vi "Read Session.vi"(8 "error in (no error)":errorcluster, 11 "Fgen PXI CFG in":refnum<class "Fgen PXI CFG.lvclass">) -> (0 "error out":errorcluster, 2 "Session":refnum<k15>, 3 "Fgen PXI CFG out":refnum<class "Fgen PXI CFG.lvclass">)   [LabVIEW 2023, in "Fgen PXI.lvlib" / "Fgen PXI CFG.lvclass"]
uses:
  Fgen PXI CFG.lvclass
  Fgen PXI CFG.lvclass/Fgen PXI CFG.ctl
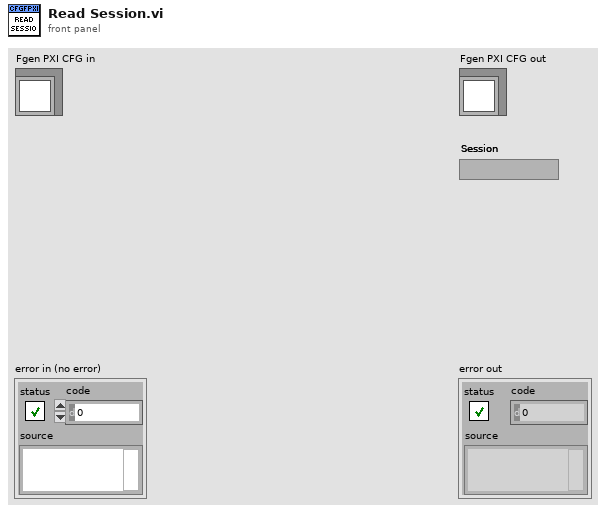
[diagram p1: front panel]
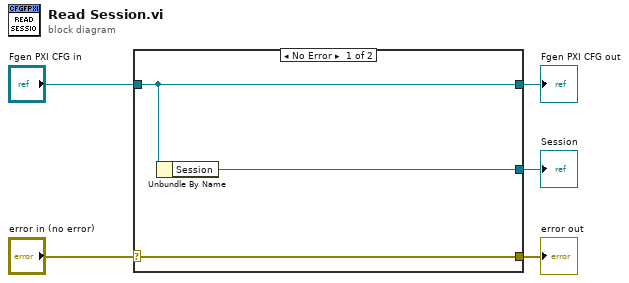
[diagram p0: block diagram]
diagram:
  n1 = case shown="No Error" "error in (no error)" {
    selector: "error in (no error)" -> [w8 w9]
    tunnel: [w8 w9] -> w4
    tunnel: [w7 w10] -> w2
    tunnel: "Fgen PXI CFG in" -> [w7 w10]
    tunnel: [w6 _] -> w1
    frame No Error {
      n2 = Unbundle By Name(w7) -> ("Session"=w6:refnum<k15>)
    }
    frame Error {
    }
  }
  "error out" <- w4
  "Fgen PXI CFG out" <- w2
  "Session" <- w1
